vi "GFITS_GetHeadTiming.vi"(9 "def_timing":string, 10 "line In":string) -> (1 "head_tim":string, 2 "line out":string)   [LabVIEW 2016]
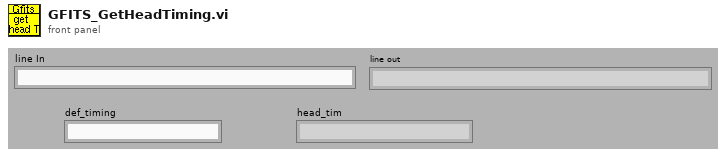
[diagram p1: front panel]
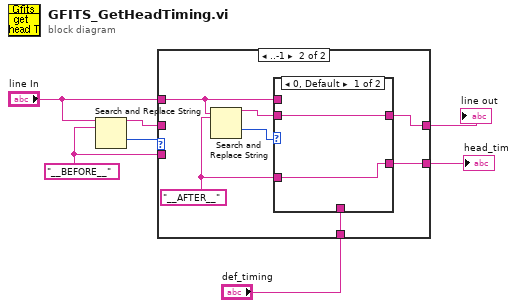
[diagram p0: block diagram]
diagram:
  w3 = "__BEFORE__" ("search string")
  n1 = Search and Replace String(input string="line In", search string=w3) -> (result string=w2:string, offset past replacement=w7:i32)  [unwired: 1 in, 7 out]
  n2 = case shown="..-1" w7 {
    tunnel: "line In" -> [_ w10]
    tunnel: "def_timing" -> [_ w15]
    tunnel: [w9 w14] -> w4
    tunnel: w3 -> [w9 _]
    tunnel: w2 -> [w8 _]
    tunnel: [w8 w11] -> w1
    frame 0, Default {
    }
    frame ..-1 {
      w13 = "__AFTER__" ("search string")
      n3 = Search and Replace String(input string=w10, search string=w13) -> (result string=w12:string, offset past replacement=w16:i32)  [unwired: 1 in, 7 out]
      n4 = case shown="0, Default" w16 {
        tunnel: w15 -> [_ w20]
        tunnel: [w18 w20] -> w14
        tunnel: w13 -> [w18 _]
        tunnel: w12 -> [w17 _]
        tunnel: [w17 w19] -> w11
        tunnel: w10 -> [_ w19]
        frame 0, Default {
        }
        frame ..-1 {
        }
      }
    }
  }
  "line out" <- w1
  "head_tim" <- w4
